vi "_New Group.vi"(8 "error in (no error)":errorcluster, 10 "Group Config":refnum<class "Group Config.lvclass">, 11 "Loop Data in":T1) -> (0 "error out":errorcluster, 2 "New Group":refnum<class "GroupAbstract.lvclass">, 3 "Loop Data":T1)   [LabVIEW 2020, in "Vecto.lvlib" / "ChannelService.lvclass"]
uses:
  ChannelService.lvclass
  ChannelService.lvclass/ChannelService.ctl
  Group Config/Group Config.lvclass
  Channel Config/Channel Config.lvclass
  GroupAbstract/GroupAbstract.lvclass
  Loop Data.ctl
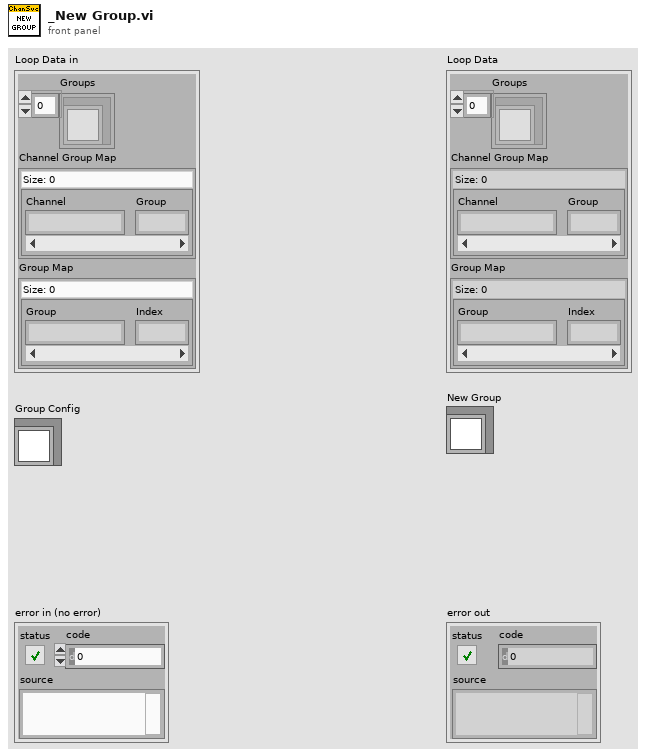
[diagram p1: front panel]
types:
  T1 = typedef "Vecto.lvlib/ChannelService.lvclass/Loop Data.ctl" = cluster{"Groups":refnum<class "GroupAbstract.lvclass">[], "Channel Group Map":map{string, i32}, "Group Map":map{string, i32}}
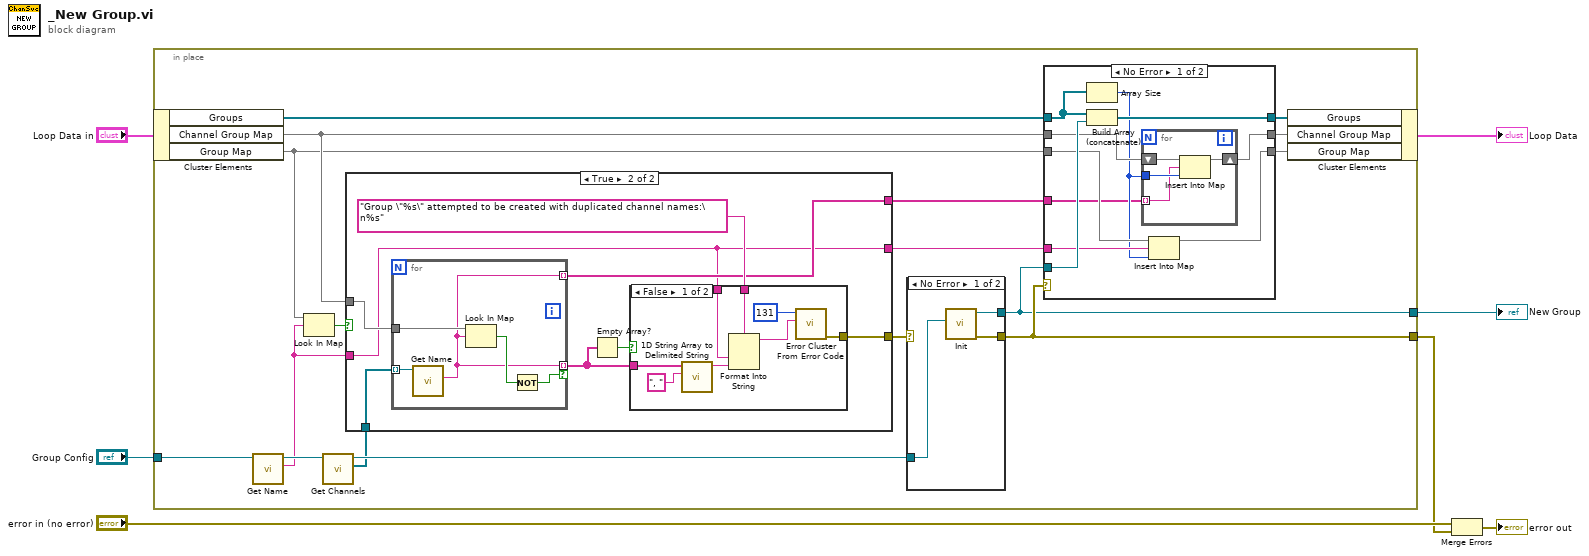
[diagram p0: block diagram]
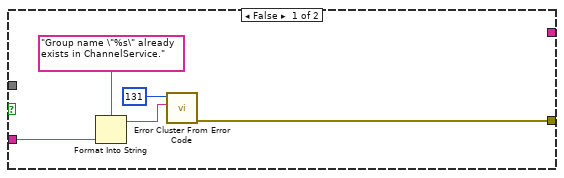
[diagram p2: hidden frame]
diagram:
  n1 = in-place {
    in-place-border: "Group Config" -> [w22]
    in-place-border: [w21] -> w4
    in-place-border: [w12] -> w2
    n2 = in-place-cluster #1("Loop Data in") -> ("Groups"=w20:refnum<class "GroupAbstract.lvclass">[], "Channel Group Map"=w18:map{string, i32}, "Group Map"=w15:map{string, i32})
    n3 = call "Get Name.vi"("Group Config in"=w22) -> ("Name"=w10:string, "Group Config out"=w11:refnum<class "Group Config.lvclass">)  [unwired: 8 in, 1 out]
    n4 = Look In Map(map=w15, key=w10) -> (key not found?=w24:bool)  [unwired: 1 in, 1 out]
    n5 = call "Get Channels.vi"("Group Config in"=w11) -> ("Channels"=w8:refnum<class "Channel Config.lvclass">[], "Group Config out"=w9:refnum<class "Group Config.lvclass">)  [unwired: 8 in, 1 out]
    n6 = case shown="True" w24 {
      tunnel: w10 -> [w28 w33]
      tunnel: w18 -> [_ w37]
      tunnel: [w25 w36] -> w23
      tunnel: [_ w34] -> w14
      tunnel: [_ w33] -> w13
      tunnel: w8 -> [_ w32]
      frame False {
        n7 = Format Into String(format string="Group name \"%s\" already exists in ChannelService.", w28) -> (resulting string=w26:string)  [unwired: 2 in, 1 out]
        n8 = call <vilib>:"Error Cluster From Error Code.vi"("error message (\"\")"=w26, "error code (0)"=131) -> ("error out"=w25:errorcluster)  [unwired: 7 in]
      }
      frame True {
        n9 = for {
          tunnel: w37 -> [w50]
          tunnel: w32 -> [w47] mode=indexing
          tunnel: [w46] -> w31 mode=indexing if=w48
          tunnel: [w46] -> w34 mode=indexing
          n10 = call "Get Name.vi"("Channel Config in"=w47) -> ("Name"=w46:string)  [unwired: 8 in, 2 out]
          n11 = Look In Map(map=w50, key=w46) -> (key not found?=w49:bool)  [unwired: 1 in, 1 out]
          n12 = Not(x=w49) -> (.not. x?=w48:bool)
        }
        n13 = Empty Array?(array=w31) -> (empty?=w30:bool)
        n14 = case shown="False" w30 {
          tunnel: [w45 _] -> w36
          tunnel: "Group \"%s\" attempted to be created with duplicated channel names:\n%s" ("format string") -> [w42 _]
          tunnel: w33 -> [w39 _]
          tunnel: w31 -> [w38 _]
          frame False {
            n15 = call <vilib>:"1D String Array to Delimited String.vi"("delimiter"=", ", "string array"=w38) -> ("delimited string"=w41:string)  [unwired: 9 in]
            n16 = Format Into String(format string=w42, w39, w41) -> (resulting string=w40:string)  [unwired: 2 in, 1 out]
            n17 = call <vilib>:"Error Cluster From Error Code.vi"("error message (\"\")"=w40, "error code (0)"=131) -> ("error out"=w45:errorcluster)  [unwired: 7 in]
          }
          frame True {
          }
        }
      }
    }
    n18 = case shown="No Error" w23 {
      selector: w23 -> [_ w71]
      tunnel: w9 -> [w68 _]
      tunnel: [w70 w71] -> w21
      tunnel: [w69 _] -> w12
      frame No Error {
        n19 = call "Init.vi"("Group Config"=w68) -> ("error out"=w70:errorcluster, "Group"=w69:refnum<class "GroupAbstract.lvclass">)  [unwired: 9 in]
      }
      frame Error {
      }
    }
    n20 = case shown="No Error" w21 {
      tunnel: w12 -> [w59 _]
      tunnel: w20 -> [w60 w67]
      tunnel: [w58 w67] -> w19
      tunnel: w18 -> [w54 w66]
      tunnel: [w51 w66] -> w17
      tunnel: [w55 w65] -> w16
      tunnel: w15 -> [w57 w65]
      tunnel: w14 -> [w52 _]
      tunnel: w13 -> [w56 _]
      frame No Error {
        n21 = Array Size(array=w60) -> (size(s)=w53:i32)
        n22 = Build Array (concatenate)(w60, w59) -> (w58:refnum<class "GroupAbstract.lvclass">[])
        n23 = for {
          shift-right: [w61] -> w51
          shift-left: w54 -> [w64]
          tunnel: w53 -> [w63]
          tunnel: w52 -> [w62] mode=indexing
          n24 = Insert Into Map(map in=w64, key=w62, value=w63) -> (map out=w61:map{string, i32})  [unwired: 2 out]
        }
        n25 = Insert Into Map(map in=w57, key=w56, value=w53) -> (map out=w55:map{string, i32})  [unwired: 2 out]
      }
      frame Error {
      }
    }
    n26 = in-place-cluster #1("Groups"=w19, "Channel Group Map"=w17, "Group Map"=w16) -> (→"Loop Data":T1)
  }
  "New Group" <- w2
  n27 = Merge Errors("error in (no error)", w4) -> (→"error out":errorcluster)
